vi "Find_Spectrometer.vi"() -> (4 "NrOfDevices":i32, 8 "AviableSpec":u8[](array[numeric]))   [LabVIEW 2020]
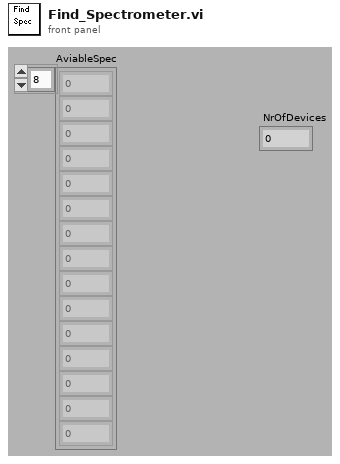
[diagram p1: front panel]
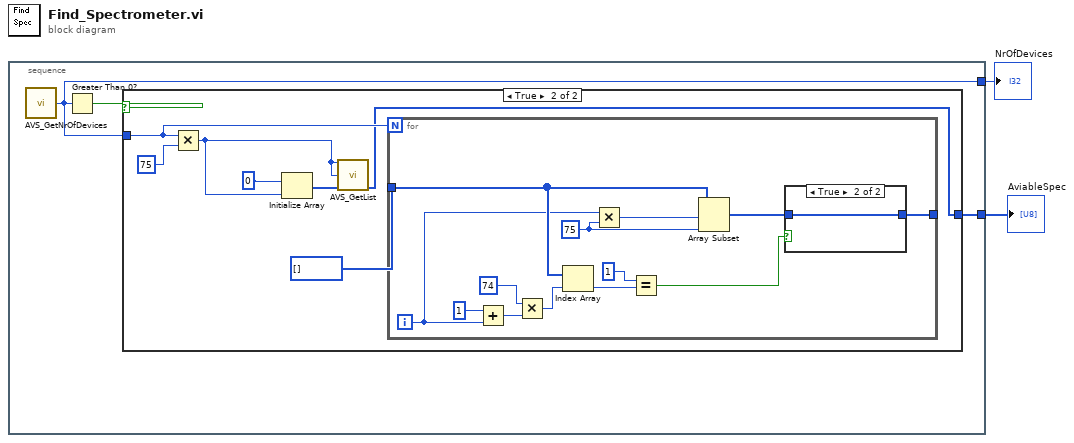
[diagram p0: block diagram]
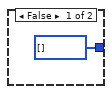
[diagram p2: hidden frame]
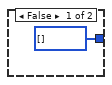
[diagram p3: hidden frame]
diagram:
  n1 = stacked-sequence {
    tunnel: [w4] -> w2
    tunnel: [w3] -> w1
    frame #0 {
      n2 = call <instrlib>:"AVS_GetNrOfDevices.vi"() -> ("Output Value"=w3:i32)  [unwired: 15 in]
      n3 = Greater Than 0?(x=w3) -> (x > 0?=w5:bool)
      n4 = case shown="True" w5 {
        tunnel: w3 -> [_ w9]
        tunnel: [u8[] [] w8] -> w4
        frame False {
        }
        frame True {
          n5 = Multiply(x=w9, y=75 ("x")) -> (x*y=w12:i32)
          n6 = Initialize Array(u8 0, w12) -> (w11:u8[])
          n7 = call <instrlib>:"AVS_GetList.vi"("ListSizeInput"=w12, "RequiredSizeInput"=w12, "ListInpit"=w11) -> ("List Output"=w8:u8[])  [unwired: 10 in, 2 out]
          n8 = for {
            N: w9 -> [_]
            tunnel: u8[] [] ("List Output") -> [w22]
            tunnel: [w16] -> _
            i -> [w15]
            w14 = 75 ("x")
            n9 = Add(x=1, y=w15) -> (x+y=w24:i32)
            n10 = Multiply(x=74, y=w24) -> (x*y=w23:i32)
            n11 = Index Array(array=w22, index=w23) -> (element=w20:u8)
            n12 = Multiply(x=w15, y=w14) -> (x*y=w26:i32)
            n13 = Equal?(x=u8 1, y=w20) -> (x = y?=w17:bool)
            n14 = Array Subset(array=w22, index=w26, length=w14) -> (w18:u8[])
            n15 = case shown="True" w17 {
              tunnel: w18 -> [_ w28]
              tunnel: [u8[] [] w28] -> w16
              frame False {
              }
              frame True {
              }
            }
          }
        }
      }
    }
  }
  "AviableSpec" <- w2
  "NrOfDevices" <- w1
